vi "SetHomeConfig.vi"(8 "error in (no error)":errorcluster, 11 "KST101 in":refnum<class "KST101.lvclass">) -> (0 "error out":errorcluster, 3 "KST101 out":refnum<class "KST101.lvclass">)   [LabVIEW 2016, in "Stepper Motor Controller.lvlib" / "KST101.lvclass"]
uses:
  KST101.lvclass
  KST101.lvclass/KST101.ctl
  D:/Workspace/ProCyteOne_LaserModuleAlignment/shared/Thorlabs/Kinesis/Dependencies/Thorlabs.MotionControl.KCube.StepperMotorCLI.dll
  Dependencies/Thorlabs.MotionControl.KCube.StepperMotorCLI.dll
  D:/Workspace/ProCyteOne_LaserModuleAlignment/shared/Thorlabs/Kinesis/Dependencies/Thorlabs.MotionControl.GenericMotorCLI.dll
  Dependencies/Thorlabs.MotionControl.GenericMotorCLI.dll
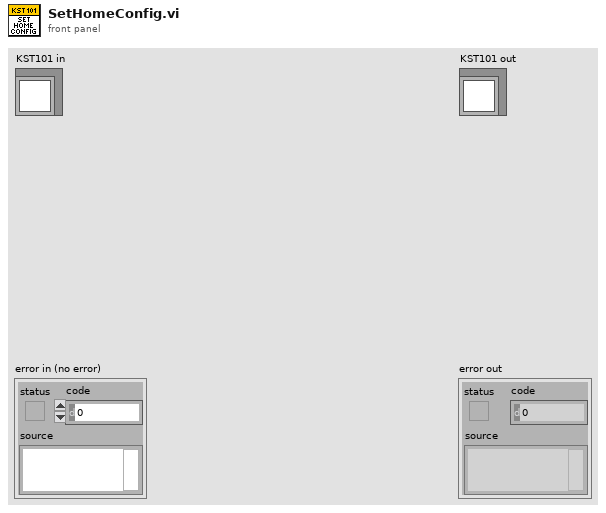
[diagram p1: front panel]
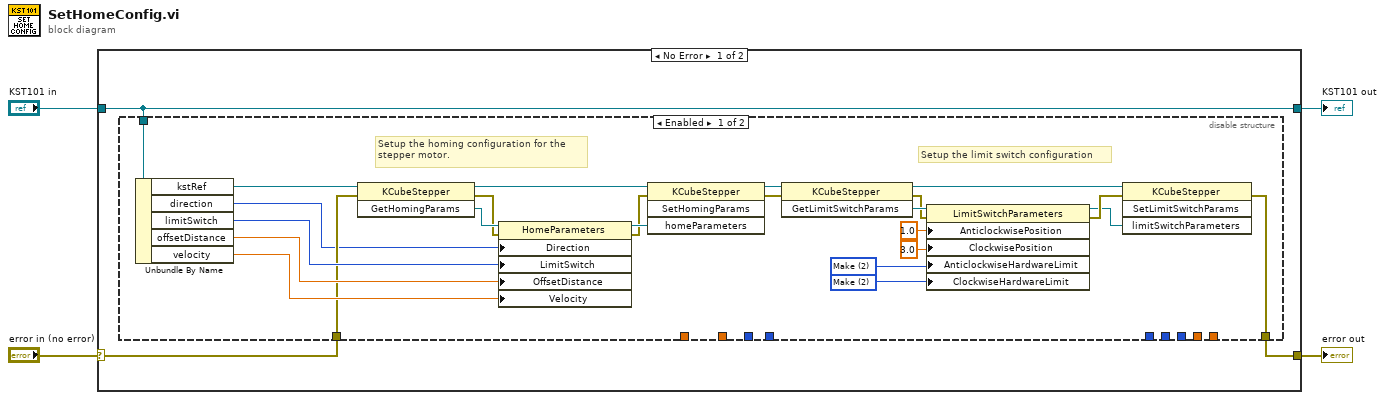
[diagram p0: block diagram]
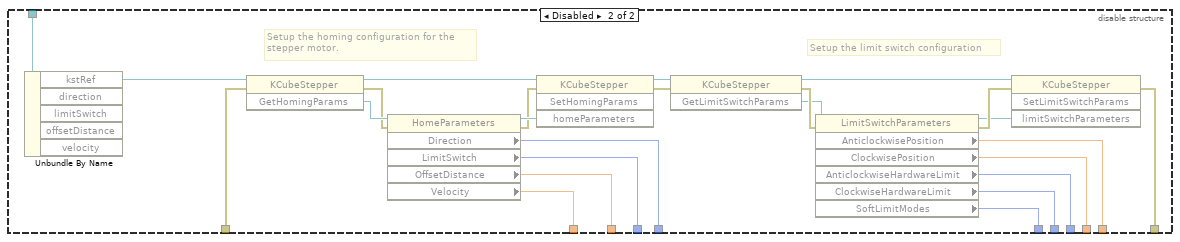
[diagram p2: hidden frame]
diagram:
  n1 = case shown="No Error" "error in (no error)" {
    selector: "error in (no error)" -> [w6 w58]
    tunnel: [w5 w58] -> w3
    tunnel: [w7 w57] -> w1
    tunnel: "KST101 in" -> [w7 w57]
    frame No Error {
      n2 = disable-structure shown="Enabled" {
        disable-tunnel: w7 -> [w31 w56]
        disable-tunnel: w6 -> [w23 w51]
        disable-tunnel: [w10 w42] -> w5
        disable-tunnel: [_ w41] -> _
        disable-tunnel: [_ w40] -> _
        disable-tunnel: [_ w39] -> _
        disable-tunnel: [_ w38] -> _
        disable-tunnel: [_ w36] -> _
        disable-tunnel: [_ w35] -> _
        disable-tunnel: [_ w34] -> _
        disable-tunnel: [_ w33] -> _
        disable-tunnel: [_ w32] -> _
        frame Enabled {
          w8 = 2 items=["Ignore"=1, "Make"=2, "Break"=3, "Home_Make"=4, "Home_Break"=5, "PMD_Index"=6, "Ignore_Swapped"=129, "Make_Swapped"=130, "Break_Swapped"=131, "Home_Make_Swapped"=132, "Home_Break_Swapped"=133] ("ClockwiseHardwareLimit")
          w9 = 2 items=["Ignore"=1, "Make"=2, "Break"=3, "Home_Make"=4, "Home_Break"=5, "PMD_Index"=6, "Ignore_Swapped"=129, "Make_Swapped"=130, "Break_Swapped"=131, "Home_Make_Swapped"=132, "Home_Break_Swapped"=133] ("AnticlockwiseHardwareLimit")
          # "Setup the limit switch configuration"
          # "Setup the homing configuration for the\nstepper motor."
          n3 = Unbundle By Name(w31) -> ("kstRef"=w20:refnum<k24>, "direction"=w22:i32, "limitSwitch"=w29:i32, "offsetDistance"=w28:dbl, "velocity"=w27:dbl)
          n4 = invoke class="KCubeStepper" method="GetHomingParams"(reference=w20, error in=w23) -> (reference out=w25:refnum<k24>, error out=w21:errorcluster, "GetHomingParams"=w24:refnum<k24>)  [unwired: 1 in]
          n5 = property class="HomeParameters"(reference=w24, error in=w21, "Direction"=w22, "LimitSwitch"=w29, "OffsetDistance"=w28, "Velocity"=w27) -> (reference out=w30:refnum<k24>, error out=w26:errorcluster)
          n6 = invoke class="KCubeStepper" method="SetHomingParams"(reference=w25, error in=w26, "homeParameters"=w30) -> (reference out=w19:refnum<k24>, error out=w18:errorcluster)  [unwired: 1 in, 2 out]
          n7 = invoke class="KCubeStepper" method="GetLimitSwitchParams"(reference=w19, error in=w18) -> (reference out=w13:refnum<k24>, error out=w14:errorcluster, "GetLimitSwitchParams"=w17:refnum<k24>)  [unwired: 1 in]
          n8 = property class="LimitSwitchParameters"(reference=w17, error in=w14, "AnticlockwisePosition"=1.0, "ClockwisePosition"=3.0, "AnticlockwiseHardwareLimit"=w9, "ClockwiseHardwareLimit"=w8) -> (reference out=w11:refnum<k24>, error out=w12:errorcluster)
          n9 = invoke class="KCubeStepper" method="SetLimitSwitchParams"(reference=w13, error in=w12, "limitSwitchParameters"=w11) -> (error out=w10:errorcluster)  [unwired: 1 in, 3 out]
        }
        frame Disabled {
          # "Setup the limit switch configuration"
          # "Setup the homing configuration for the\nstepper motor."
          n10 = Unbundle By Name(w56) -> ("kstRef"=w49:refnum<k24>)  [unwired: 4 out]
          n11 = invoke class="KCubeStepper" method="GetHomingParams"(reference=w49, error in=w51) -> (reference out=w53:refnum<k24>, error out=w50:errorcluster, "GetHomingParams"=w52:refnum<k24>)  [unwired: 1 in]
          n12 = property class="HomeParameters"(reference=w52, error in=w50) -> (reference out=w55:refnum<k24>, error out=w54:errorcluster, "Direction"=w41:i32, "LimitSwitch"=w40:i32, "OffsetDistance"=w39:dbl, "Velocity"=w38:dbl)
          n13 = invoke class="KCubeStepper" method="SetHomingParams"(reference=w53, error in=w54, "homeParameters"=w55) -> (reference out=w48:refnum<k24>, error out=w47:errorcluster)  [unwired: 1 in, 2 out]
          n14 = invoke class="KCubeStepper" method="GetLimitSwitchParams"(reference=w48, error in=w47) -> (reference out=w45:refnum<k24>, error out=w46:errorcluster, "GetLimitSwitchParams"=w37:refnum<k24>)  [unwired: 1 in]
          n15 = property class="LimitSwitchParameters"(reference=w37, error in=w46) -> (reference out=w43:refnum<k24>, error out=w44:errorcluster, "AnticlockwisePosition"=w36:dbl, "ClockwisePosition"=w35:dbl, "AnticlockwiseHardwareLimit"=w34:i32, "ClockwiseHardwareLimit"=w33:i32, "SoftLimitModes"=w32:i32)
          n16 = invoke class="KCubeStepper" method="SetLimitSwitchParams"(reference=w45, error in=w44, "limitSwitchParameters"=w43) -> (error out=w42:errorcluster)  [unwired: 1 in, 3 out]
        }
      }
    }
    frame Error {
    }
  }
  "error out" <- w3
  "KST101 out" <- w1
